vi "BRig_Host__Loop_Consumer_RunState__closedLoop_parseOutput2_cmd_subunit1.vi"(11 "String":string) -> (2 "output_cmd":u16[](array[numeric]), 3 "output_cmd":bool)   [LabVIEW 2014]
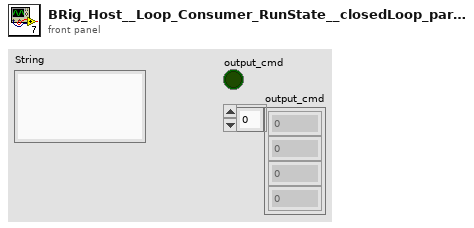
[diagram p1: front panel]
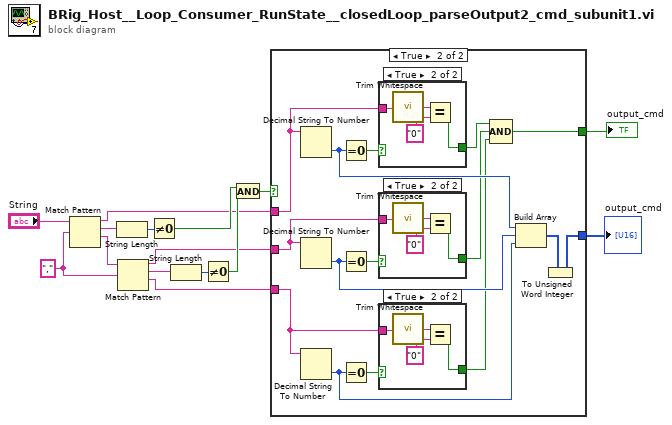
[diagram p0: block diagram]
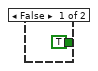
[diagram p3: hidden frame]
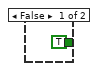
[diagram p4: hidden frame]
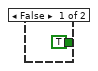
[diagram p5: hidden frame]
diagram:
  w11 = "," ("regular expression")
  n1 = Match Pattern(string="String", regular expression=w11) -> (before substring=w5:string, match substring=w13:string, after substring=w12:string)  [unwired: 1 in, 1 out]
  n2 = String Length(string=w13) -> (length=w15:i32)
  n3 = Match Pattern(string=w12, regular expression=w11) -> (before substring=w4:string, match substring=w9:string, after substring=w3:string)  [unwired: 1 in, 1 out]
  n4 = Not Equal To 0?(x=w15) -> (x != 0?=w7:bool)
  n5 = String Length(string=w9) -> (length=w10:i32)
  n6 = Not Equal To 0?(x=w10) -> (x != 0?=w8:bool)
  n7 = And(x=w7, y=w8) -> (x .and. y?=w6:bool)
  n8 = case shown="True" w6 {
    tunnel: w5 -> [_ w29]
    tunnel: w4 -> [_ w22]
    tunnel: w3 -> [_ w19]
    tunnel: [_ w24] -> w2
    tunnel: [_ w16] -> w1
    frame False {
    }
    frame True {
      n9 = Decimal String To Number(string=w29) -> (number=w27:i32)  [unwired: 2 in, 1 out]
      n10 = Decimal String To Number(string=w22) -> (number=w25:i32)  [unwired: 2 in, 1 out]
      n11 = Decimal String To Number(string=w19) -> (number=w26:i32)  [unwired: 2 in, 1 out]
      n12 = Equal To 0?(x=w27) -> (x = 0?=w30:bool)
      n13 = Equal To 0?(x=w25) -> (x = 0?=w23:bool)
      n14 = Equal To 0?(x=w26) -> (x = 0?=w20:bool)
      n15 = case shown="True" w30 {
        tunnel: w29 -> [_ w43]
        tunnel: [TRUE w45] -> w28
        frame False {
        }
        frame True {
          n16 = call <vilib>:"Trim Whitespace.vi"("string"=w43) -> ("trimmed string"=w42:string)  [unwired: 1 in]
          n17 = Equal?(x=w42, y="0" ("x")) -> (x = y?=w45:bool)
        }
      }
      n18 = case shown="True" w23 {
        tunnel: w22 -> [_ w38]
        tunnel: [TRUE w40] -> w21
        frame False {
        }
        frame True {
          n19 = call <vilib>:"Trim Whitespace.vi"("string"=w38) -> ("trimmed string"=w37:string)  [unwired: 1 in]
          n20 = Equal?(x=w37, y="0" ("x")) -> (x = y?=w40:bool)
        }
      }
      n21 = case shown="True" w20 {
        tunnel: w19 -> [_ w33]
        tunnel: [TRUE w35] -> w18
        frame False {
        }
        frame True {
          n22 = call <vilib>:"Trim Whitespace.vi"("string"=w33) -> ("trimmed string"=w32:string)  [unwired: 1 in]
          n23 = Equal?(x=w32, y="0" ("x")) -> (x = y?=w35:bool)
        }
      }
      n24 = Compound Arithmetic op=AND(w28, w21, w18) -> (w24:bool)
      n25 = Build Array(w27, w25, w26) -> (w17:i32[])
      n26 = To Unsigned Word Integer(number=w17) -> (unsigned 16bit integer=w16:u16[])
    }
  }
  "output_cmd" <- w2
  "output_cmd" <- w1
